vi "myANPR RT.vi"() -> ()   [LabVIEW 2014]
uses:
  <vilib>/userdefined/High Color/IMAQdx.ctl
  <vilib>/vision/driver/NI_Vision_Acquisition_Software.lvlib
panel:
  in  "Stop Button":bool
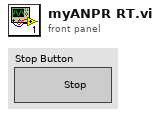
[diagram p1: front panel]
types:
  T1 = typedef "IMAQdx.ctl" = refnum<k21>
  T2 = typedef "Image Type" = u32
  T3 = typedef "IMAQ Image.ctl" = refnum<image>
  T4 = cluster{"Global Rectangle":cluster{"x1Left":i32, "y1Top":i32, "x2Right":i32, "y2Bottom":i32}, "Centroid":cluster{"x":sgl, "y":sgl}, "Object Size":u32, "Score":dbl}[]
  T5 = typedef "ROI Descriptor" = cluster{"Global Rectangle":i32[], "Contours":cluster{"ID":enum32{"External", "Internal"}, "Type":u32, "Coordinates":i32[]}[]}
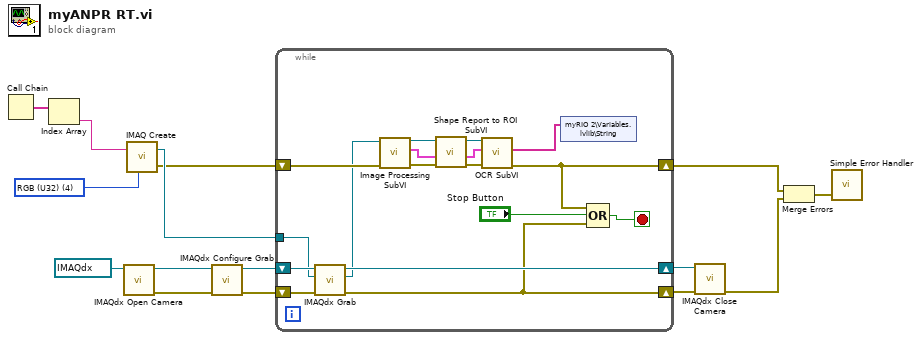
[diagram p0: block diagram]
diagram:
  w13 = T2 4 items=["Grayscale (U8)", "Grayscale (I16)", "Grayscale (SGL)", "Complex (CSG)", "RGB (U32)", "HSL (U32)", "RGB (U64)", "Grayscale (U16)"] ("Image Type")
  n1 = Call Chain() -> (call chain=w15:string[])
  n2 = Index Array(array=w15) -> (element=w14:string)  [unwired: 1 in]
  n3 = call <vilib>:"IMAQdx Open Camera.vi"("Session In"=T1 "cam0") -> ("error out"=w11:errorcluster, "Session Out"=w12:T1)  [unwired: 9 in]
  n4 = call "IMAQ Create"("Image Name"=w14, "Image Type"=w13) -> ("New Image"=w6:T3, "error out"=w5:errorcluster)  [unwired: 2 in, 1 out]
  n5 = call <vilib>:"IMAQdx Configure Grab.vi"("error in"=w11, "Session In"=w12) -> ("error out"=w9:errorcluster, "Session Out"=w10:T1)  [unwired: 8 in]
  n6 = while {
    shift-right: [w16] -> w3
    shift-left: w5 -> [w26]
    shift-right: [w23] -> w8
    shift-left: w10 -> [w25]
    shift-right: [w20] -> w7
    shift-left: w9 -> [w24]
    tunnel: w6 -> [w19]
    stop <- w22 stop-if-true
    n7 = call <vilib>:"IMAQdx Grab.vi"("error in"=w24, "Image In"=w19, "Session In"=w25) -> ("error out"=w20:errorcluster, "Image Out"=w18:T3, "Session Out"=w23:T1)  [unwired: 5 in, 1 out]
    n8 = call "Image Processing SubVI.vi"("Error In"=w26, "Image Refnum In"=w18) -> ("Error Out"=w27:errorcluster, "Shape Report"=w30:T4, "Image Refnum Out"=w32:T3)  [unwired: 7 in]
    n9 = call "Shape Report to ROI SubVI.vi"("Image In"=w32, "Shape Report"=w30, "Error In"=w27) -> ("Image Out"=w31:T3, "ROI Array Within Image"=w29:T5[], "Error Out"=w28:errorcluster)  [unwired: 5 in]
    n10 = call "OCR SubVI.vi"("error in (no error)"=w28, "ROI Array Within Image"=w29, "Refnum in"=w31) -> ("error out"=w16:errorcluster, "Read String"=w17:string[])  [unwired: 6 in, 1 out]
    n11 = shared-variable "myRIO 2\\Variables.lvlib\\String"(w17) -> ()  [unwired: 1 in, 1 out]
    n12 = Compound Arithmetic op=OR(w16, "Stop Button", w20) -> (w22:bool)
  }
  n13 = call <vilib>:"IMAQdx Close Camera.vi"("error in"=w7, "Session In"=w8) -> ("error out"=w2:errorcluster)  [unwired: 9 in]
  n14 = Merge Errors(w3, w2) -> (w4:errorcluster)
  n15 = call <vilib>:"Simple Error Handler.vi"("error in (no error)"=w4) -> ()  [unwired: 4 in, 5 out]
